vi "Count Balls.vi"(10 "Reset Ball Count?":bool, 11 "Mode":enum16{"Init", "Run", "End"}(ring)=enum."Run") -> (1 "Top Sensor?":bool, 2 "Bottom Back?":bool, 3 "Number Of Balls":i32)   [LabVIEW 2011]
uses:
  TypeDefs/Digital Module 1.ctl
  <vilib>/Rock Robotics/SystemInterfaces/Typedef/FPGA_TypedefDigitalModule.ctl
  <vilib>/Rock Robotics/SystemInterfaces/DIO/FPGA_DIOChannel.ctl
  Team Code/Robot Global Data.vi
panel:
  in  "Digital Module A":T1={"Module"=enum."Digital Module 1", "Left Enc A"=enum."DIO 1", "Left Enc B"=enum."DIO 2", "Right Enc A"=enum."DIO 3", "Right Enc B"=enum."DIO 4", "Outer Sensor"=enum."DIO 5", "Inner Sensor"=enum."DIO 6", "Upper Sensor"=enum."DIO 7", "Shooter Tachometer"=enum."DIO 8", "Unassigned"=enum."DIO 9", "Unassigned"=enum."DIO 10", "Top Conveyer Sensor"=enum."DIO 11", "Arm Upper Limit"=enum."DIO 12", "Arm Lower Limit"=enum."DIO 13", "1510"=enum."DIO 14"}
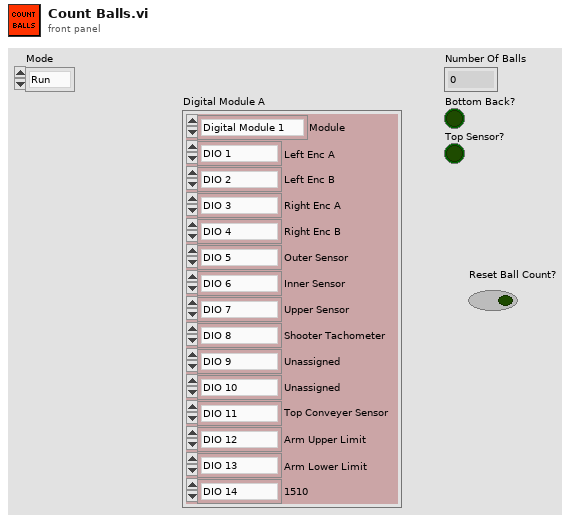
[diagram p1: front panel]
types:
  T1 = typedef "Digital Module 1.ctl" = cluster{"Module":T2, "Left Enc A":T3, "Left Enc B":T3, "Right Enc A":T3, "Right Enc B":T3, "Outer Sensor":T3, "Inner Sensor":T3, "Upper Sensor":T3, "Shooter Tachometer":T3, "Unassigned":T3, "Unassigned":T3, "Top Conveyer Sensor":T3, "Arm Upper Limit":T3, "Arm Lower Limit":T3, "1510":T3}
  T2 = typedef "FPGA_TypedefDigitalModule.ctl" = enum16{"Digital Module 1", "Digital Module 2"}
  T3 = typedef "FPGA_DIOChannel.ctl" = enum8{"DIO 1", "DIO 2", "DIO 3", "DIO 4", "DIO 5", "DIO 6", "DIO 7", "DIO 8", "DIO 9", "DIO 10", "DIO 11", "DIO 12", "DIO 13", "DIO 14", "Invalid"}
  T4 = typedef "WPI_DigitalInputDevRef.ctl" = cluster{"DevStatus":errorcluster, "DIO Channel":T3, "Digital Module":T2}
  T5 = cluster{"Ball Count Up":bool, "Ball Count Down":bool}
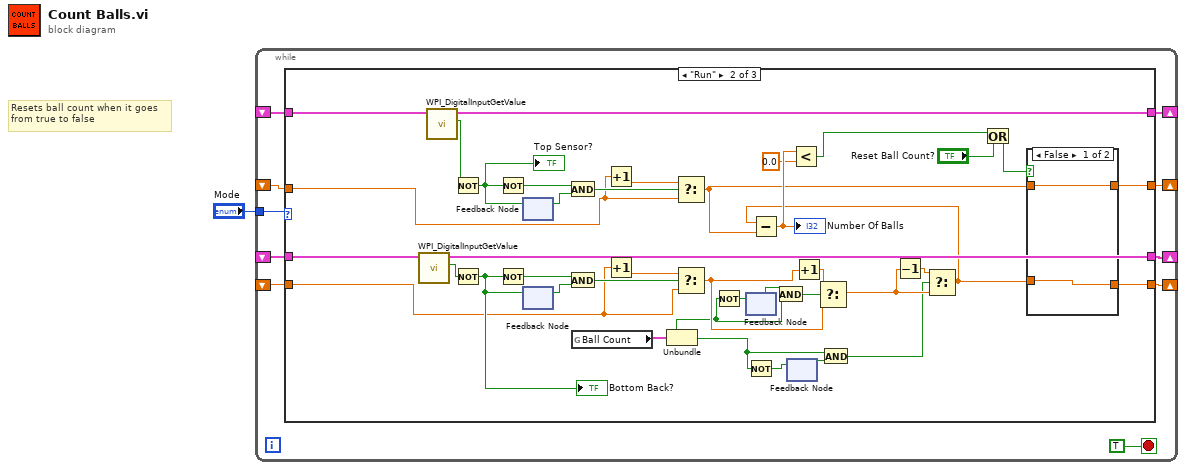
[diagram p0: block diagram]
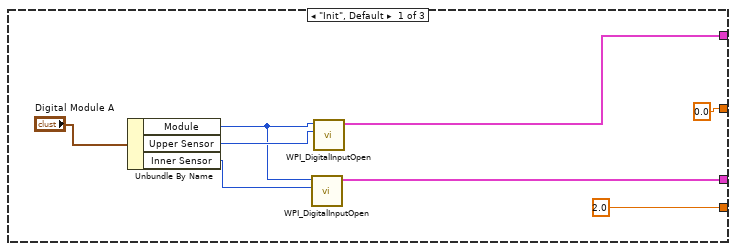
[diagram p2: hidden frame]
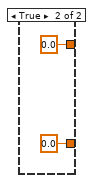
[diagram p3: hidden frame]
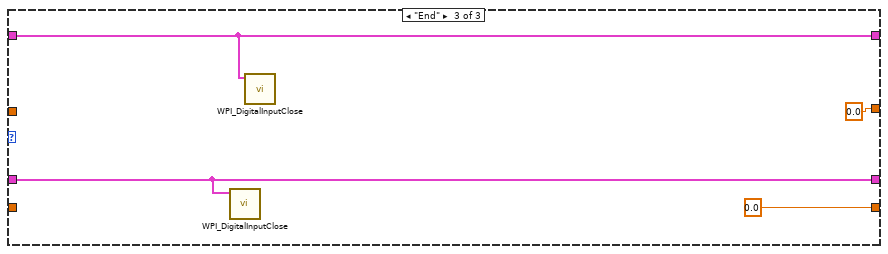
[diagram p4: hidden frame]
diagram:
  # "Resets ball count when it goes\nfrom true to false"
  n1 = while {
    tunnel: "Mode" -> [w10]
    shift-right: [w9] -> _
    shift-left: _ -> [w6]
    shift-right: [w8] -> _
    shift-left: _ -> [w7]
    shift-right: [w5] -> _
    shift-left: _ -> [w4]
    shift-right: [w3] -> _
    shift-left: _ -> [w2]
    stop <- TRUE stop-if-true
    n2 = case shown="\"Run\"" w10 {
      tunnel: [w15 w59 w66] -> w9
      tunnel: [w13 w41 w64] -> w8
      tunnel: w7 -> [_ w30 w64]
      tunnel: w6 -> [_ w29 w66]
      tunnel: [2.0 w23 0.0] -> w5
      tunnel: w4 -> [_ w27 _]
      tunnel: [0.0 w25 0.0] -> w3
      tunnel: w2 -> [_ w28 _]
      frame "Init", Default {
        n3 = Unbundle By Name("Digital Module A") -> ("Module"=w17:T2, "Upper Sensor"=w18:T3, "Inner Sensor"=w16:T3)
        n4 = call <vilib>:"WPI_DigitalInputOpen.vi"("DIO Channel"=w16, "Digital Module (Module 1)"=w17) -> ("DigitalInputDevRef"=w15:T4)  [unwired: 8 in, 1 out]
        n5 = call <vilib>:"WPI_DigitalInputOpen.vi"("DIO Channel"=w18, "Digital Module (Module 1)"=w17) -> ("DigitalInputDevRef"=w13:T4)  [unwired: 8 in, 1 out]
      }
      frame "Run" {
        n6 = call <vilib>:"WPI_DigitalInputGetValue.vi"("DigitalInputDevRef"=w29) -> ("Value"=w43:bool, "DigitalInputDevRef"=w59:T4)  [unwired: 8 in, 1 out]
        n7 = call <vilib>:"WPI_DigitalInputGetValue.vi"("DigitalInputDevRef"=w30) -> ("Value"=w36:bool, "DigitalInputDevRef"=w41:T4)  [unwired: 8 in, 1 out]
        n8 = Not(x=w36) -> (.not. x?=w20:bool)
        "Top Sensor?" <- w20
        n9 = Not(x=w43) -> (.not. x?=w42:bool)
        "Bottom Back?" <- w42
        n10 = Not(x=w20) -> (.not. x?=w37:bool)
        n11 = Not(x=w42) -> (.not. x?=w44:bool)
        n12 = feedback #1() -> (w40:bool)  [unwired: 1 in]
        n13 = feedback-in #1(w20) -> ()
        n14 = feedback-in #2(w42) -> ()
        n15 = feedback #2() -> (w58:bool)  [unwired: 1 in]
        n16 = And(x=w37, y=w40) -> (x .and. y?=w39:bool)
        n17 = And(x=w44, y=w58) -> (x .and. y?=w57:bool)
        n18 = global read "Robot Global Data.vi" "Ball Count"() -> (w55:T5)
        n19 = Increment(x=w28) -> (x+1=w38:dbl)
        n20 = Increment(x=w27) -> (x+1=w56:dbl)
        n21 = Unbundle(w55) -> ("Ball Count Up"=w35:bool, "Ball Count Down"=w46:bool)
        n22 = Select(t=w38, s=w39, f=w28) -> (s? t:f=w26:dbl)
        n23 = Select(t=w56, s=w57, f=w27) -> (s? t:f=w51:dbl)
        n24 = Not(x=w35) -> (.not. x?=w54:bool)
        n25 = feedback-in #3(w54) -> ()
        n26 = feedback #3() -> (w34:bool)  [unwired: 1 in]
        n27 = Not(x=w46) -> (.not. x?=w47:bool)
        n28 = And(x=w34, y=w35) -> (x .and. y?=w53:bool)
        n29 = feedback #4() -> (w48:bool)  [unwired: 1 in]
        n30 = feedback-in #4(w47) -> ()
        n31 = Increment(x=w51) -> (x+1=w52:dbl)
        n32 = Select(t=w52, s=w53, f=w51) -> (s? t:f=w49:dbl)
        n33 = And(x=w46, y=w48) -> (x .and. y?=w45:bool)
        n34 = Decrement(x=w49) -> (x-1=w50:dbl)
        n35 = Select(t=w50, s=w45, f=w49) -> (s? t:f=w24:dbl)
        n36 = Subtract(x=w24, y=w26) -> (x-y=w33:dbl)
        "Number Of Balls" <- w33
        n37 = Less?(x=w33, y=0.0) -> (x < y?=w21:bool)
        n38 = Or(x=w21, y="Reset Ball Count?") -> (x .or. y?=w22:bool)
        n39 = case shown="False" w22 {
          tunnel: w24 -> [w61 _]
          tunnel: [w61 0.0] -> w23
          tunnel: w26 -> [w60 _]
          tunnel: [w60 0.0] -> w25
          frame False {
          }
          frame True {
          }
        }
      }
      frame "End" {
        n40 = call <vilib>:"WPI_DigitalInputClose.vi"("DigitalInputDevRef"=w66) -> ()  [unwired: 10 in, 1 out]
        n41 = call <vilib>:"WPI_DigitalInputClose.vi"("DigitalInputDevRef"=w64) -> ()  [unwired: 10 in, 1 out]
      }
    }
  }
